vi "MH_GetDLLPath.vi"(9 "DllName_32bit":string, 10 "PathToDLL":path, 11 "DllName_64bit":string) -> (2 "file exists?":bool, 3 "DLLPath":path)   [LabVIEW 2019]
uses:
  <vilib>/Utility/sysdir.llb/System Directory Type.ctl
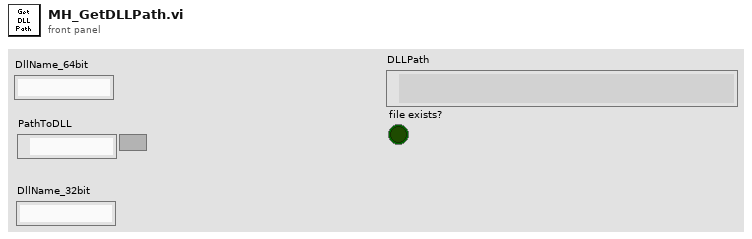
[diagram p1: front panel]
types:
  T1 = typedef "System Directory Type.ctl" = i32
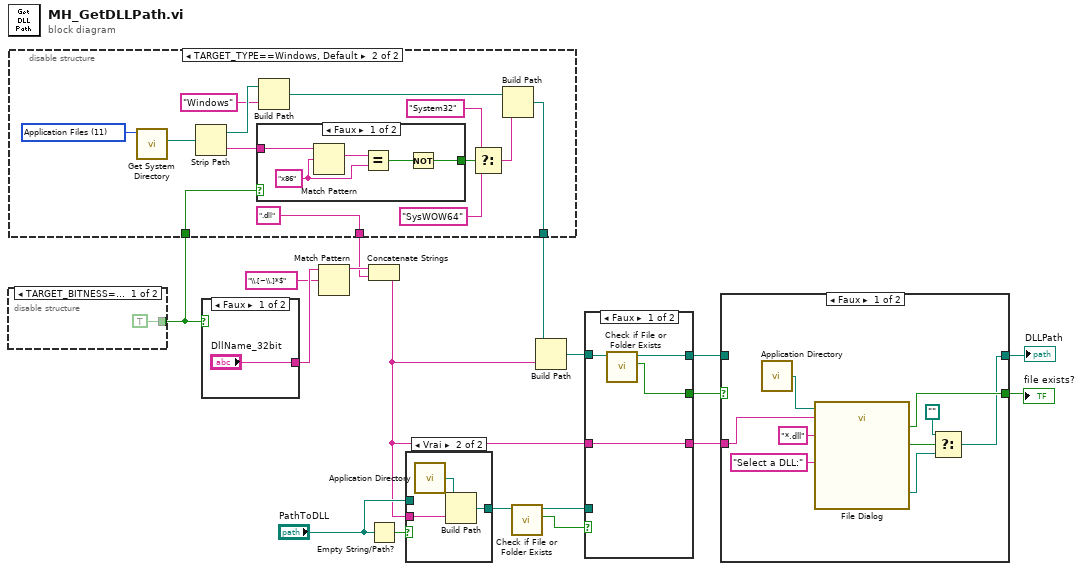
[diagram p0: block diagram]
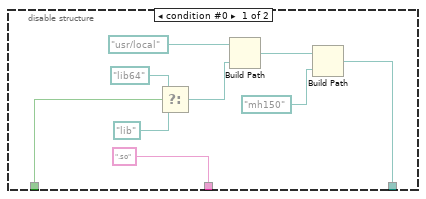
[diagram p2: hidden frame]
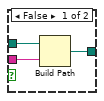
[diagram p5: hidden frame]
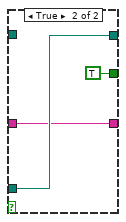
[diagram p6: hidden frame]
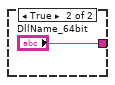
[diagram p7: hidden frame]
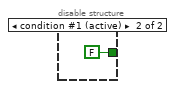
[diagram p8: hidden frame]
diagram:
  n1 = disable-structure shown="TARGET_BITNESS==64, Default" {
    disable-tunnel: [TRUE FALSE] -> w8
    frame condition #0 {
    }
    frame condition #1 (active) {
    }
  }
  n2 = disable-structure shown="TARGET_TYPE==Windows, Default" {
    disable-tunnel: w8 -> [w29 w32]
    disable-tunnel: [w22 w31] -> w7
    disable-tunnel: [".so" ".dll"] -> w1
    frame condition #0 {
      n3 = Select(t=path "lib64" ("appended path"), s=w29, f=path "lib" ("appended path")) -> (s? t:f=w25:path)
      n4 = Build Path(base path=path "usr/local" ("appended path"), name or relative path=w25) -> (appended path=w24:path)
      n5 = Build Path(base path=w24, name or relative path=path "mh150" ("appended path")) -> (appended path=w22:path)
    }
    frame condition #1 (active) {
      w41 = T1 11 items=["User Home"=0, "User Desktop"=1, "User Documents"=2, "User Application Data"=3, "User Preferences"=4, "User Temporary"=5, "Public Documents"=6, "Public Application Data"=7, "Public Preferences"=8, "Public Cache"=13, "System Core Libraries"=9, "System Installed Libraries"=10, "Application Files"=11, "Boot Volume Root"=12] ("system directory type")
      n6 = call <vilib>:"Get System Directory.vi"("system directory type"=w41) -> ("system directory"=w42:path)  [unwired: 10 in]
      n7 = Strip Path(path=w42) -> (stripped path=w40:path, name=w38:string)
      n8 = case shown="Faux" w32 {
        selector: w32 -> [_ w48]
        tunnel: [w43 w48] -> w35
        tunnel: w38 -> [w47 _]
        frame False {
          w46 = "x86" ("regular expression")
          n9 = Match Pattern(string=w47, regular expression=w46) -> (match substring=w45:string)  [unwired: 1 in, 3 out]
          n10 = Equal?(x=w45, y=w46) -> (x = y?=w44:bool)
          n11 = Not(x=w44) -> (.not. x?=w43:bool)
        }
        frame True {
        }
      }
      n12 = Build Path(base path=w40, name or relative path="Windows") -> (appended path=w33:path)
      n13 = Select(t="System32" ("name or relative path"), s=w35, f="SysWOW64" ("name or relative path")) -> (s? t:f=w34:string)
      n14 = Build Path(base path=w33, name or relative path=w34) -> (appended path=w31:path)
    }
  }
  n15 = case shown="Faux" w8 {
    tunnel: ["DllName_32bit" "DllName_64bit"] -> w5
    frame False {
    }
    frame True {
    }
  }
  n16 = Match Pattern(string=w5, regular expression="\\.[~\\.]*$") -> (before substring=w3:string)  [unwired: 4 out]
  n17 = Concatenate Strings(w3, w1) -> (w2:string)
  n18 = Empty String/Path?(string/path="PathToDLL") -> (empty?=w16:bool)
  n19 = case shown="Vrai" w16 {
    tunnel: "PathToDLL" -> [w53 _]
    tunnel: w2 -> [w52 w55]
    tunnel: [w51 w54] -> w14
    frame False {
      n20 = Build Path(base path=w53, name or relative path=w52) -> (appended path=w51:path)
    }
    frame True {
      n21 = call <vilib>:"Application Directory.vi"() -> ("Application Directory"=w56:path)
      n22 = Build Path(base path=w56, name or relative path=w55) -> (appended path=w54:path)
    }
  }
  n23 = call <vilib>:"Check if File or Folder Exists.vi"("path"=w14) -> ("file or folder exists?"=w18:bool, "dup path"=w17:path)  [unwired: 8 in, 1 out]
  n24 = Build Path(base path=w7, name or relative path=w2) -> (appended path=w6:path)
  n25 = case shown="Faux" w18 {
    tunnel: w6 -> [w60 _]
    tunnel: [w59 TRUE ("file or folder exists?")] -> w13
    tunnel: [w58 w63] -> w12
    tunnel: w17 -> [_ w63]
    tunnel: [w57 w61] -> w9
    tunnel: w2 -> [w57 w61]
    frame False {
      n26 = call <vilib>:"Check if File or Folder Exists.vi"("path"=w60) -> ("file or folder exists?"=w59:bool, "dup path"=w58:path)  [unwired: 8 in, 1 out]
    }
    frame True {
    }
  }
  n27 = case shown="Faux" w13 {
    selector: w13 -> [_ w73]
    tunnel: w12 -> [_ w74]
    tunnel: [w65 w74] -> w11
    tunnel: [w68 w73] -> w10
    tunnel: w9 -> [w71 _]
    frame False {
      n28 = call <vilib>:"Application Directory.vi"() -> ("Application Directory"=w72:path)
      n29 = call "File Dialog"("start path"=w72, "prompt"="Select a DLL:", "default name"=w71, "pattern (all files)"="*.dll") -> ("selected path"=w66:path, "exists"=w68:bool, "cancelled"=w67:bool)  [unwired: 8 in, 1 out]
      n30 = Select(t=path "", s=w67, f=w66) -> (s? t:f=w65:path)
    }
    frame True {
    }
  }
  "DLLPath" <- w11
  "file exists?" <- w10
